vi "calculator.vi"() -> ()   [LabVIEW 2010]
panel:
  in  "CLC":bool
  out "Numeric":dbl
  in  "=":bool
  out "oper":string[](array[string])
  out "num_array":dbl[](array[numeric])
  out "number":i32
  in  "stop 2":bool
  in  "/":bool
  in  "*":bool
  in  "-":bool
  in  "+":bool
  out "Show":string
  in  "stop":bool
  in  "0":bool
  in  "9":bool
  in  "8":bool
  in  "7":bool
  in  "6":bool
  in  "5":bool
  in  "4":bool
  in  "3":bool
  in  "2":bool
  in  "1":bool
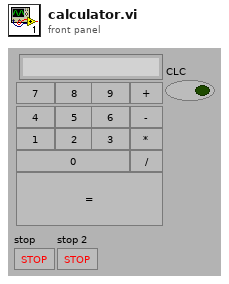
[diagram p1: front panel]
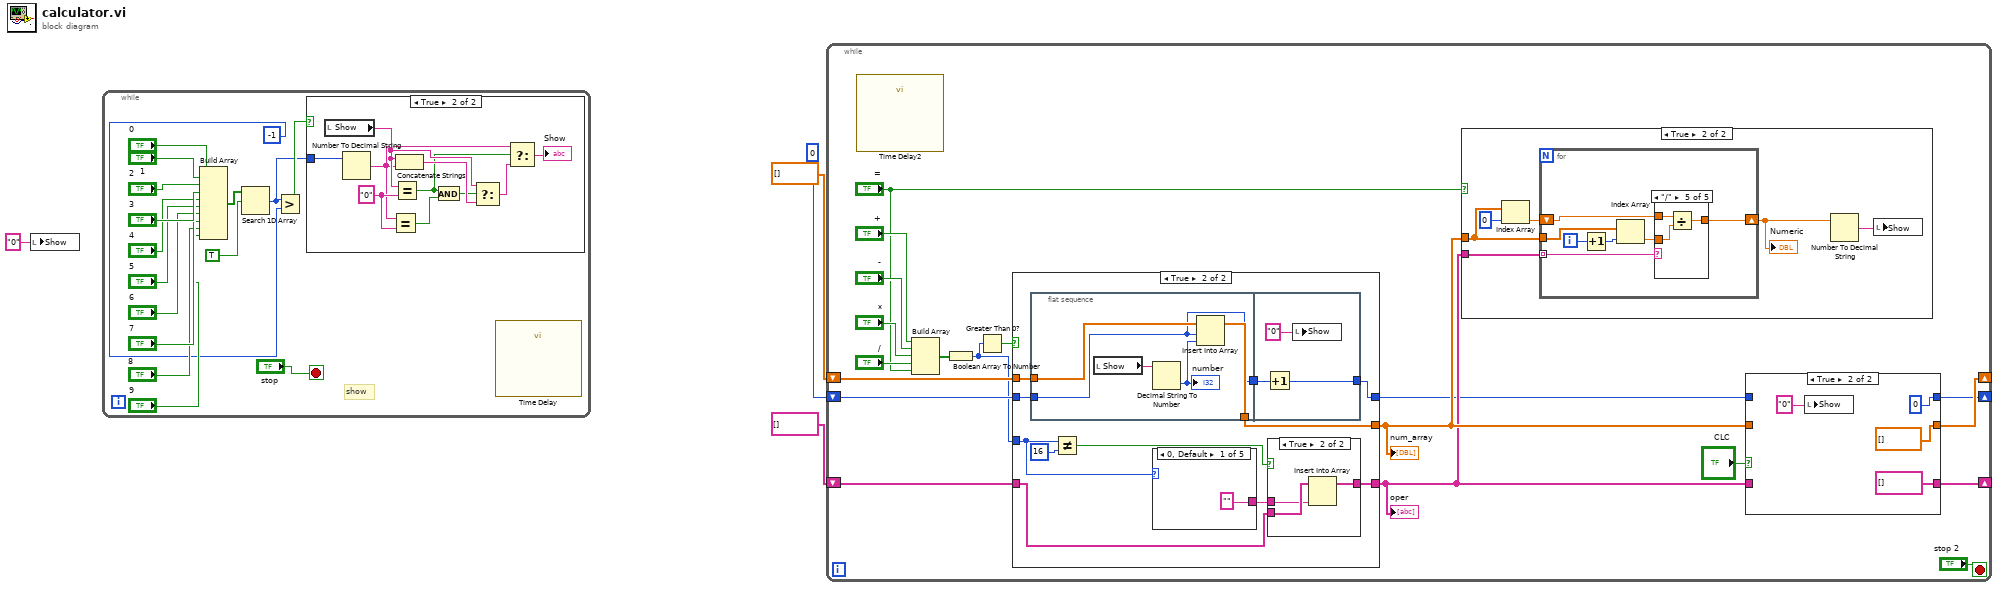
[diagram p0: block diagram]
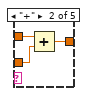
[diagram p5: hidden frame]
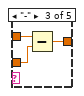
[diagram p6: hidden frame]
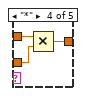
[diagram p7: hidden frame]
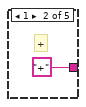
[diagram p10: hidden frame]
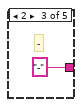
[diagram p11: hidden frame]
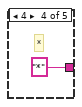
[diagram p12: hidden frame]
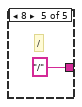
[diagram p13: hidden frame]
diagram:
  n1 = local write "Show"("0" ("String")) -> ()
  n2 = while {
    stop <- "stop" stop-if-true
    # "show"
    n3 = Build Array("0", "1", "2", "3", "4", "5", "6", "7", "8", "9") -> (w9:bool[])
    n4 = Search 1D Array(1D array=w9, element=TRUE) -> (index of element=w5:i32)  [unwired: 1 in]
    n5 = Greater?(x=w5, y=-1) -> (0:w6:bool)
    n6 = case shown="True" w6 {
      tunnel: w5 -> [_ w30]
      frame False {
      }
      frame True {
        w27 = "0" ("y")
        n7 = local read "Show"() -> (w28:string)
        n8 = Number To Decimal String(number=w30) -> (decimal integer string=w23:string)  [unwired: 1 in]
        n9 = Equal?(x=w23, y=w27) -> (x = y?=w26:bool)
        n10 = Equal?(x=w28, y=w27) -> (x = y?=w24:bool)
        n11 = Concatenate Strings(w28, w23) -> (w29:string)
        n12 = And(x=w24, y=w26) -> (x .and. y?=w25:bool)
        n13 = Select(t=w28, s=w25, f=w29) -> (s? t:f=w22:string)
        n14 = Select(t=w23, s=w24, f=w22) -> (s? t:f=→"Show":string)
      }
    }
    n15 = call "Time Delay"() -> ()  [unwired: 11 in, 1 out]
  }
  n16 = while {
    shift-right: [w37] -> _
    shift-left: dbl[] [] -> [w42]
    shift-right: [w32] -> _
    shift-left: 0 -> [w41]
    shift-right: [w34] -> _
    shift-left: string[] [] -> [w40]
    stop <- "stop 2" stop-if-true
    n17 = call "Time Delay2"() -> ()  [unwired: 11 in, 1 out]
    n18 = Build Array("+", "-", "*", "/", "=") -> (w44:bool[])
    n19 = Boolean Array To Number(Boolean array=w44) -> (number=w39:u32)
    n20 = Greater Than 0?(x=w39) -> (x > 0?=w43:bool)
    n21 = case shown="True" w43 {
      tunnel: w42 -> [w84 w95]
      tunnel: [w84 w94] -> w36
      tunnel: w41 -> [w83 w93]
      tunnel: [w83 w91] -> w33
      tunnel: w39 -> [_ w86]
      tunnel: w40 -> [w82 w90]
      tunnel: [w82 w88] -> w35
      frame False {
      }
      frame True {
        n22 = flat-sequence {
          tunnel: w95 -> [w108]
          tunnel: [w107] -> w94
          tunnel: w93 -> [w105]
          tunnel: [w105] -> w92
          tunnel: w92 -> [w111]
          tunnel: [w110] -> w91
          frame #0 {
            n23 = local read "Show"() -> (w109:string)
            n24 = Decimal String To Number(string=w109) -> (number=w106:i32)  [unwired: 2 in, 1 out]
            "number" <- w106
            n25 = Insert Into Array(array=w108, index=w105, new element=w106) -> (w107:dbl[])
          }
          frame #1 {
            n26 = Increment(x=w111) -> (x+1=w110:i32)
            n27 = local write "Show"("0" ("String")) -> ()
          }
        }
        n28 = Not Equal?(x=w86, y=u32 16) -> (x != y?=w87:bool)
        n29 = case shown="0, Default" w86 {
          tunnel: ["" "+" "-" "*" "/"] -> w89
          frame 0, Default {
          }
          frame 1 {
            # "+"
          }
          frame 2 {
            # "-"
          }
          frame 4 {
            # "*"
          }
          frame 8 {
            # "/"
          }
        }
        n30 = case shown="True" w87 {
          tunnel: w90 -> [w96 w99]
          tunnel: w89 -> [_ w98]
          tunnel: [w96 w97] -> w88
          frame False {
          }
          frame True {
            n31 = Insert Into Array(array=w99, new element=w98) -> (w97:string[])  [unwired: 1 in]
          }
        }
      }
    }
    "num_array" <- w36
    "oper" <- w35
    n32 = case shown="True" "=" {
      tunnel: w36 -> [_ w61]
      tunnel: w35 -> [_ w62]
      frame False {
      }
      frame True {
        n33 = Index Array(array=w61, index=0) -> (element=w59:dbl)
        n34 = for {
          tunnel: w62 -> [w69] mode=indexing
          tunnel: w61 -> [w68]
          shift-right: [w64] -> w58
          shift-left: w59 -> [w63]
          i -> [w67]
          n35 = Increment(x=w67) -> (x+1=w66:i32)
          n36 = Index Array(array=w68, index=w66) -> (element=w65:dbl)
          n37 = case shown="\"/\"" w69 {
            tunnel: w65 -> [_ w72 w74 w77 w80]
            tunnel: [_ w71 w73 w76 w79] -> w64
            tunnel: w63 -> [_ w70 w75 w78 w81]
            frame "False", Default {
            }
            frame "+" {
              n38 = Add(x=w70, y=w72) -> (x+y=w71:dbl)
            }
            frame "-" {
              n39 = Subtract(x=w75, y=w74) -> (x-y=w73:dbl)
            }
            frame "*" {
              n40 = Multiply(x=w78, y=w77) -> (x*y=w76:dbl)
            }
            frame "/" {
              n41 = Divide(x=w81, y=w80) -> (x/y=w79:dbl)
            }
          }
        }
        "Numeric" <- w58
        n42 = Number To Decimal String(number=w58) -> (decimal integer string=w57:string)  [unwired: 1 in]
        n43 = local write "Show"(w57) -> ()
      }
    }
    n44 = case shown="True" "CLC" {
      tunnel: [w52 dbl[] []] -> w37
      tunnel: w36 -> [w52 _]
      tunnel: w35 -> [w51 _]
      tunnel: [w51 string[] []] -> w34
      tunnel: w33 -> [w50 _]
      tunnel: [w50 0] -> w32
      frame False {
      }
      frame True {
        n45 = local write "Show"("0" ("String")) -> ()
      }
    }
  }
